vi "ShowTimer.vi"() -> ()   [LabVIEW 2020, in "Analyze.lvlib" / "Analyze Timer.lvclass"]
uses:
  Analyze Timer.lvclass
  <vilib>/Utility/miscctls.llb/LVRectTypeDef.ctl
  Utility/POLARIS Vision utility.lvlib
panel:
  in  "Font:Size":u32=80
  in  "Panel Bounds":T1
  in  "Color Box":u32(colorbox)=15663143
  in  "stop":bool
  out "error out":errorcluster
  in  "Notifier":refnum<notifier>
  out "Timer":i32
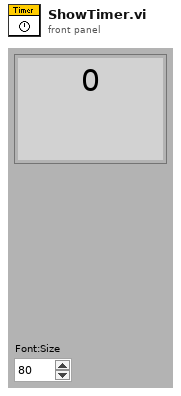
[diagram p1: front panel]
types:
  T1 = typedef "LVRectTypeDef.ctl" = cluster{"Left":i16, "Top":i16, "Right":i16, "Bottom":i16}
  T2 = typedef "eventvkey.ctl" = enum16{"ASCII", "Enter", "Return", "Shift", "Ctrl", "Alt", "Cmd", "Opt", "Caps", "NumLock", "Clear", "Break", "Up", "Down", "Left", "Right", "Insert", "Delete", "Home", "End", "PageUp", "PageDown", "Escape", "Help", "Pause", "ScrollLock", "F1", "F2", "F3", "F4", "F5", "F6", "F7", "F8", "F9", "F10", "F11", "F12", "F13", "F14", "F15", "F16", "F17", "F18", "F19", "F20", "F21", "F22", "F23", "F24", "Play", "VolumeUp", "VolumeDown", "Mute", "Two Byte Char"}
  T3 = cluster{"Shift":bool, "Ctrl":bool, "Alt":bool, "Cmd":bool, "Opt":bool}
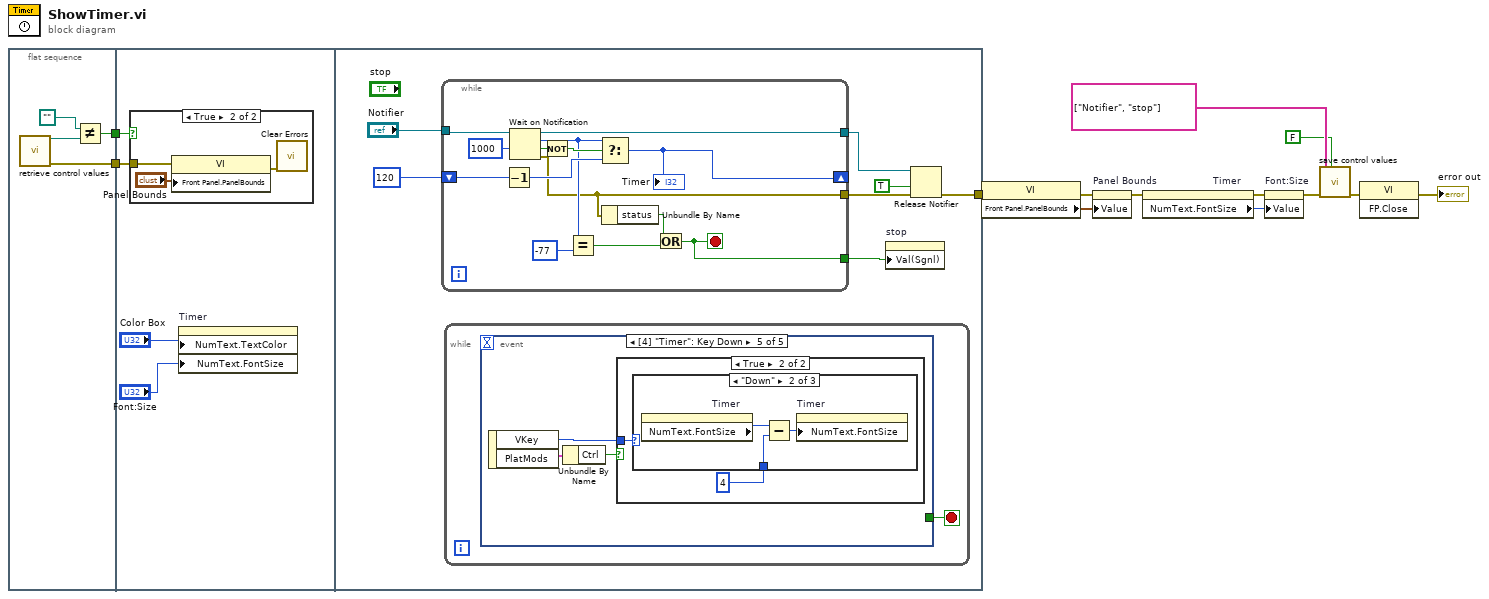
[diagram p0: block diagram]
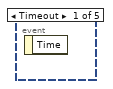
[diagram p3: hidden frame]
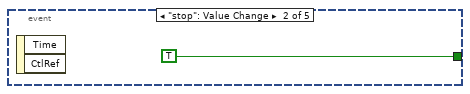
[diagram p4: hidden frame]
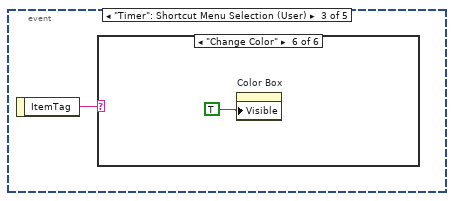
[diagram p5: hidden frame]
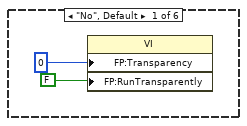
[diagram p6: hidden frame]
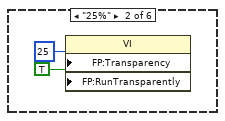
[diagram p7: hidden frame]
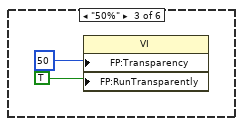
[diagram p8: hidden frame]
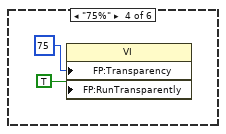
[diagram p9: hidden frame]
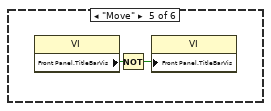
[diagram p10: hidden frame]
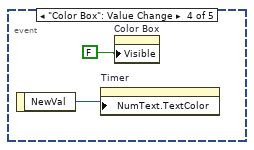
[diagram p11: hidden frame]
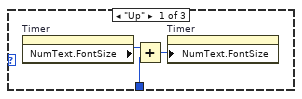
[diagram p13: hidden frame]
diagram:
  n1 = flat-sequence {
    tunnel: [w17] -> w7
    tunnel: [w14] -> w5
    tunnel: w7 -> [w20]
    tunnel: w5 -> [w19]
    tunnel: [w25] -> w10
    frame #0 {
      n2 = call "retrieve control values.vi"() -> ("error out"=w17:errorcluster, "path out"=w16:path)  [unwired: 10 in]
      n3 = Not Equal?(x=path "", y=w16) -> (x != y?=w14:bool)
    }
    frame #1 {
      n4 = case shown="True" w19 {
        tunnel: w20 -> [_ w23]
        frame False {
        }
        frame True {
          n5 = property class="VI"(error in=w23, "Front Panel.PanelBounds"="Panel Bounds") -> (error out=w22:errorcluster)  [unwired: 1 in, 1 out]
          n6 = call <vilib>:"Clear Errors.vi"("error in (no error)"=w22) -> ()  [unwired: 5 in, 2 out]
        }
      }
      n7 = property on="Timer" class="DigNum (strict)"("NumText.TextColor"="Color Box", "NumText.FontSize"="Font:Size") -> ()  [unwired: 2 in, 2 out]
    }
    frame #2 {
      n8 = while {
        tunnel: "Notifier" -> [w45]
        shift-right: [w39] -> _
        shift-left: 120 -> [w42]
        tunnel: [w36] -> w29
        tunnel: [w34] -> w28
        tunnel: [w32] -> w26
        stop <- w32 stop-if-true
        n9 = Decrement(x=w42) -> (x-1=w41:i32)
        n10 = Wait on Notification(notifier=w45, timeout in ms (-1)=1000) -> (notifier out=w34:refnum<notifier>, notification=w38:i32, timed out?=w43:bool, error out=w36:errorcluster)  [unwired: 2 in]
        n11 = Not(x=w43) -> (.not. x?=w40:bool)
        n12 = Equal?(x=w38, y=-77) -> (x = y?=w33:bool)
        n13 = Select(t=w38, s=w40, f=w41) -> (s? t:f=w39:i32)
        "Timer" <- w39
        n14 = Unbundle By Name(w36) -> ("status"=w35:bool)
        n15 = Or(x=w35, y=w33) -> (x .or. y?=w32:bool)
      }
      n16 = while {
        stop <- w46 stop-if-true
        n17 = event shown="[4] \"Timer\": Key Down" {
          selector: _ -> [_ _ _ _ _]
          dyn-events: _ -> [_ _ _ _ _]
          timeout: _ -> [_ _ _ _ _]
          tunnel: [_ TRUE _ _ _] -> w46
          event Timeout {
            n18 = event-data() -> ()  [unwired: 1 in, 1 out]
          }
          event "stop": Value Change {
            n19 = event-data() -> ()  [unwired: 1 in, 2 out]
          }
          event "Timer": Shortcut Menu Selection (User) {
            n20 = event-data() -> ("ItemTag"=w48:string)  [unwired: 1 in]
            n21 = case shown="\"Change Color\"" w48 {
              frame "No", Default {
                n22 = property class="VI"("FP:Transparency"=u8 0 ("Front Panel Window:Transparency"), "FP:RunTransparently"=FALSE ("Front Panel Window:Run VI Transparently")) -> ()  [unwired: 2 in, 2 out]
              }
              frame "25%" {
                n23 = property class="VI"("FP:Transparency"=u8 25 ("Front Panel Window:Transparency"), "FP:RunTransparently"=TRUE ("Front Panel Window:Run VI Transparently")) -> ()  [unwired: 2 in, 2 out]
              }
              frame "50%" {
                n24 = property class="VI"("FP:Transparency"=u8 50 ("Front Panel Window:Transparency"), "FP:RunTransparently"=TRUE ("Front Panel Window:Run VI Transparently")) -> ()  [unwired: 2 in, 2 out]
              }
              frame "75%" {
                n25 = property class="VI"("FP:Transparency"=u8 75 ("Front Panel Window:Transparency"), "FP:RunTransparently"=TRUE ("Front Panel Window:Run VI Transparently")) -> ()  [unwired: 2 in, 2 out]
              }
              frame "Move" {
                n26 = property class="VI"() -> ("Front Panel.TitleBarVis"=w58:bool)  [unwired: 2 in, 2 out]
                n27 = Not(x=w58) -> (.not. x?=w57:bool)
                n28 = property class="VI"("Front Panel.TitleBarVis"=w57) -> ()  [unwired: 2 in, 2 out]
              }
              frame "Change Color" {
                n29 = property on="Color Box" class="ColBox"("Visible"=TRUE) -> ()  [unwired: 2 in, 2 out]
              }
            }
          }
          event "Color Box": Value Change {
            n30 = event-data() -> ("NewVal"=w61:u32)  [unwired: 1 in]
            n31 = property on="Timer" class="DigNum (strict)"("NumText.TextColor"=w61) -> ()  [unwired: 2 in, 2 out]
            n32 = property on="Color Box" class="ColBox"("Visible"=FALSE) -> ()  [unwired: 2 in, 2 out]
          }
          event "Timer": Key Down {
            n33 = event-data() -> ("VKey"=w63:T2, "PlatMods"=w64:T3)  [unwired: 1 in]
            n34 = Unbundle By Name(w64) -> ("Ctrl"=w62:bool)
            n35 = case shown="True" w62 {
              tunnel: w63 -> [_ w66]
              frame False {
              }
              frame True {
                n36 = case shown="\"Down\"" w66 {
                  tunnel: u32 4 ("x") -> [w67 w70 _]
                  frame "Up" {
                    n37 = property on="Timer" class="DigNum (strict)"() -> ("NumText.FontSize"=w69:u32)  [unwired: 2 in, 2 out]
                    n38 = Add(x=w69, y=w67) -> (x+y=w68:u32)
                    n39 = property on="Timer" class="DigNum (strict)"("NumText.FontSize"=w68) -> ()  [unwired: 2 in, 2 out]
                  }
                  frame "Down" {
                    n40 = property on="Timer" class="DigNum (strict)"() -> ("NumText.FontSize"=w72:u32)  [unwired: 2 in, 2 out]
                    n41 = Subtract(x=w72, y=w70) -> (x-y=w71:u32)
                    n42 = property on="Timer" class="DigNum (strict)"("NumText.FontSize"=w71) -> ()  [unwired: 2 in, 2 out]
                  }
                  frame "Left", Default {
                  }
                }
              }
            }
          }
        }
      }
      n43 = property on="stop" class="Bool (strict)"("Val(Sgnl)"=w26) -> ()  [unwired: 2 in, 2 out]
      n44 = Release Notifier(notifier=w28, force destroy? (F)=TRUE, error in (no error)=w29) -> (error out=w25:errorcluster)  [unwired: 2 out]
    }
  }
  n45 = property class="VI"(error in=w10) -> (error out=w8:errorcluster, "Front Panel.PanelBounds"=w9:T1)  [unwired: 1 in, 1 out]
  n46 = property on="Panel Bounds" class="Clust (strict)"(error in=w8, "Value"=w9) -> (error out=w4:errorcluster)  [unwired: 1 in, 1 out]
  n47 = property on="Timer" class="DigNum (strict)"(error in=w4) -> (error out=w3:errorcluster, "NumText.FontSize"=w1:u32)  [unwired: 1 in, 1 out]
  n48 = property on="Font:Size" class="DigNum (strict)"(error in=w3, "Value"=w1) -> (error out=w2:errorcluster)  [unwired: 1 in, 1 out]
  n49 = call "save control values.vi"("Append timestamp (true)"=FALSE, "error in"=w2, "Dont save"=string[] ["Notifier", "stop"]) -> ("error out"=w12:errorcluster)  [unwired: 5 in, 1 out]
  n50 = invoke class="VI" method="FP.Close"(error in=w12) -> (error out=→"error out":errorcluster)  [unwired: 2 in, 2 out]
